vi "Is Home.vi"(8 "error in (no error)":errorcluster, 9 "timeout in ms (0)":i32, 11 "Cylinder in":refnum<class "Cylinder.lvclass">) -> (0 "error out":errorcluster, 1 "timed out?":bool, 2 "Cylinder is Home":bool, 3 "Cylinder out":refnum<class "Cylinder.lvclass">)   [LabVIEW 2015, in "cRIO-Carbondioxide.lvlib" / "CO2-Actor.lvlib" / "Cylinder.lvclass"]
uses:
  Cylinder.lvclass
  Cylinder.lvclass/Cylinder.ctl
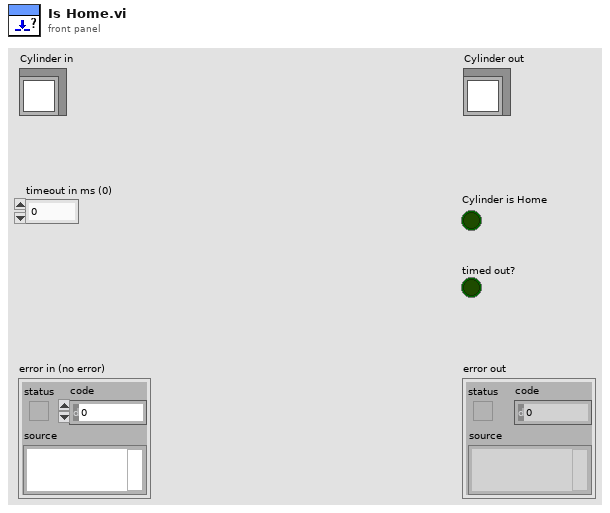
[diagram p1: front panel]
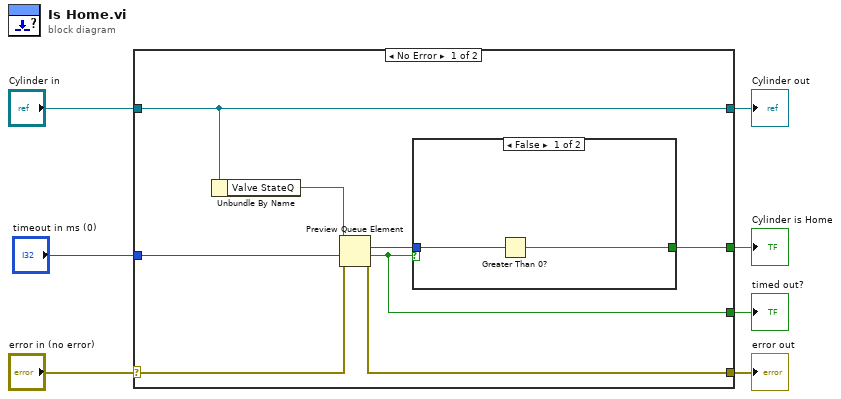
[diagram p0: block diagram]
diagram:
  n1 = case shown="No Error" "error in (no error)" {
    selector: "error in (no error)" -> [w13 w19]
    tunnel: [w12 w19] -> w6
    tunnel: [w15 w18] -> w4
    tunnel: "Cylinder in" -> [w15 w18]
    tunnel: [w11 _] -> w3
    tunnel: [w9 _] -> w2
    tunnel: "timeout in ms (0)" -> [w8 _]
    frame No Error {
      n2 = Unbundle By Name(w15) -> ("Valve StateQ"=w14:refnum<queue>)
      n3 = Preview Queue Element(queue=w14, timeout in ms (-1)=w8, error in (no error)=w13) -> (element=w10:u16, timed out?=w9:bool, error out=w12:errorcluster)  [unwired: 1 out]
      n4 = case shown="False" w9 {
        tunnel: [w16 _] -> w11
        tunnel: w10 -> [w17 _]
        frame False {
          n5 = Greater Than 0?(x=w17) -> (x > 0?=w16:bool)
        }
        frame True {
        }
      }
    }
    frame Error {
    }
  }
  "error out" <- w6
  "Cylinder out" <- w4
  "Cylinder is Home" <- w3
  "timed out?" <- w2
